vi "Initialize.vi"(8 "error in (no error)":errorcluster, 11 "Core Plugin User Interface in":refnum<class "Core Plugin User Interface.lvclass">) -> (0 "error out":errorcluster, 3 "Core Plugin User Interface out":refnum<class "Core Plugin User Interface.lvclass">)   [LabVIEW 2020, in "DSF Core.lvlib" / "Core Plugin User Interface.lvclass"]
uses:
  Core Plugin User Interface.lvclass
  C:/Users/nitest/Desktop/Git/niveristand-data-sharing-framework-custom-device/Source/Core/Classes/User Interface/User Interface.lvclass
  Configuration/Core/Plugin/Plugin Configuration.lvclass
  C:/Users/nitest/Desktop/Git/niveristand-data-sharing-framework-custom-device/Source/Core/Classes/Configuration/Configuration.lvclass
  User Interface.lvclass
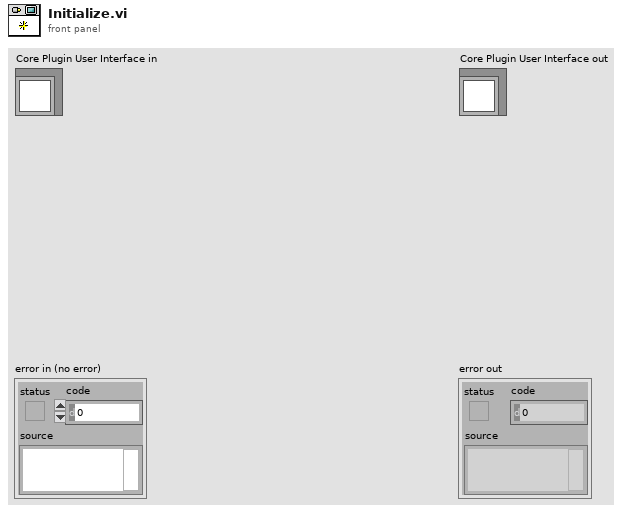
[diagram p1: front panel]
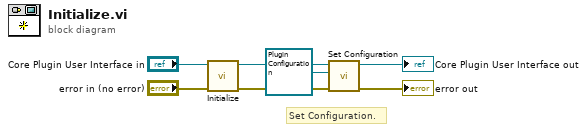
[diagram p0: block diagram]
diagram:
  # "Set Configuration."
  n1 = call-parent "Initialize.vi"("error in (no error)"="error in (no error)", "User Interface in"="Core Plugin User Interface in") -> ("error out"=w1:errorcluster, "User Interface out"=w2:refnum<class "Core Plugin User Interface.lvclass">)  [unwired: 8 in]
  n2 = call "Set Configuration.vi"("error in (no error)"=w1, "configuration"=refnum<class "Plugin Configuration.lvclass"> refnum ("DSF Core.lvlib:Plugin Configuration.lvclass"), "User Interface in"=w2) -> ("error out"=→"error out":errorcluster, "User Interface out"=→"Core Plugin User Interface out":refnum<class "Core Plugin User Interface.lvclass">)  [unwired: 7 in]
